vi "Alert.vi"(7 "Mode":T1(ring), 8 "error in (no error)":errorcluster, 10 "Queue In":cluster{"Certificate":bool, "Card Info":string}={"Certificate"=TRUE, "Card Info"=""}) -> (0 "error out":errorcluster, 2 "Queue Out":cluster{"Certificate":bool, "Card Info":string}={"Certificate"=TRUE, "Card Info"=""})   [LabVIEW 2011]
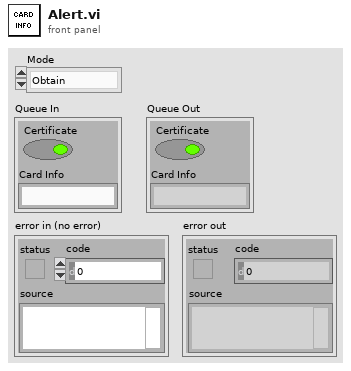
[diagram p1: front panel]
types:
  T1 = enum16{"Obtain", "Enqueue", "Dequeue", "Release"}
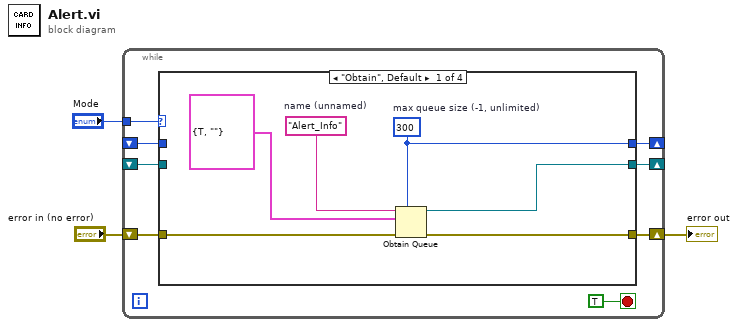
[diagram p0: block diagram]
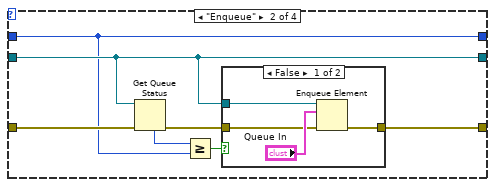
[diagram p2: hidden frame]
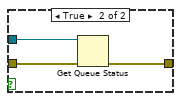
[diagram p3: hidden frame]
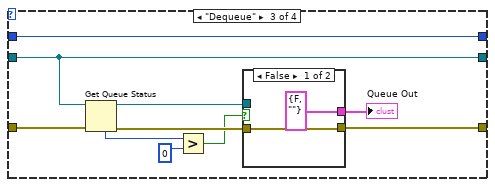
[diagram p4: hidden frame]
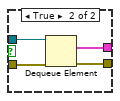
[diagram p5: hidden frame]
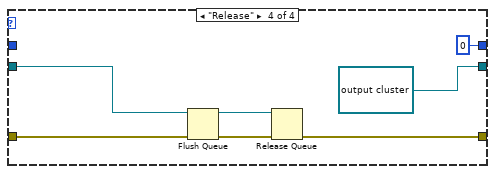
[diagram p6: hidden frame]
diagram:
  n1 = while {
    tunnel: "Mode" -> [w11]
    shift-right: [w9] -> w1
    shift-left: "error in (no error)" -> [w10]
    shift-right: [w8] -> _
    shift-left: _ -> [w7]
    shift-right: [w5] -> _
    shift-left: _ -> [w4]
    stop <- TRUE stop-if-true
    n2 = case shown="\"Obtain\", Default" w11 {
      tunnel: w10 -> [w17 w23 w40 w49]
      tunnel: [w16 w24 w41 w54] -> w9
      tunnel: [w14 w19 w38 refnum<queue> refnum ("queue out")] -> w8
      tunnel: w7 -> [_ w19 w38 w53]
      tunnel: [w12 w18 w32 0 ("max queue size (-1, unlimited)")] -> w5
      tunnel: w4 -> [_ w18 w32 _]
      frame "Obtain", Default {
        w12 = 300  # max queue size (-1, unlimited)
        w15 = "Alert_Info"  # name (unnamed)
        n3 = Obtain Queue(max queue size (-1, unlimited)=w12, name (unnamed)=w15, element data type=cluster{"Certificate":bool, "Card Info":string} {"Certificate"=TRUE, "Card Info"=""} ("output cluster"), error in (no error)=w17) -> (queue out=w14:refnum<queue>, error out=w16:errorcluster)  [unwired: 1 in, 1 out]
      }
      frame "Enqueue" {
        n4 = Get Queue Status(queue=w19, error in (no error)=w23) -> (error out=w22:errorcluster, # elements in queue=w21:i32)  [unwired: 1 in, 6 out]
        n5 = Greater Or Equal?(x=w21, y=w18) -> (x >= y?=w20:bool)
        n6 = case shown="False" w20 {
          tunnel: [w28 w29] -> w24
          tunnel: w22 -> [w26 w30]
          tunnel: w19 -> [w25 w31]
          frame False {
            n7 = Enqueue Element(queue=w25, element="Queue In", error in (no error)=w26) -> (error out=w28:errorcluster)  [unwired: 1 in, 2 out]
          }
          frame True {
            n8 = Get Queue Status(queue=w31, error in (no error)=w30) -> (error out=w29:errorcluster)  [unwired: 1 in, 7 out]
          }
        }
      }
      frame "Dequeue" {
        n9 = Get Queue Status(queue=w38, error in (no error)=w40) -> (queue out=w37:refnum<queue>, error out=w39:errorcluster, # elements in queue=w35:i32)  [unwired: 1 in, 5 out]
        n10 = Greater?(x=w35, y=0) -> (0:w34:bool)
        n11 = case shown="False" w34 {
          tunnel: [w43 w47] -> w41
          tunnel: [cluster{"Certificate":bool, "Card Info":string} {"Certificate"=FALSE, "Card Info"=""} ("output cluster") w46] -> w33
          tunnel: w39 -> [w43 w45]
          tunnel: w37 -> [_ w44]
          frame False {
          }
          frame True {
            n12 = Dequeue Element(queue=w44, error in (no error)=w45) -> (element=w46:cluster{"Certificate":bool, "Card Info":string}, error out=w47:errorcluster)  [unwired: 1 in, 2 out]
          }
        }
        "Queue Out" <- w33
      }
      frame "Release" {
        n13 = Flush Queue(queue=w53, error in (no error)=w49) -> (queue out=w50:refnum<queue>, error out=w48:errorcluster)  [unwired: 1 out]
        n14 = Release Queue(queue=w50, error in (no error)=w48) -> (error out=w54:errorcluster)  [unwired: 1 in, 2 out]
      }
    }
  }
  "error out" <- w1
